vi "Create IResultHandler.vi"(8 "error in (no error)":errorcluster, 11 "IWampMessage":refnum<class "IWampMessage.lvclass">) -> (0 "error out":errorcluster, 3 "IResultHandler":refnum<class "IResultHandler.lvclass">)   [LabVIEW 2020, in "wamplv.lvlib"]
uses:
  wamplv.lvlib
  SerialisedMessages/JSONMessage/WampMessage JSON.lvclass
  SerialisedMessages/MsgPackMessage/WampMessage MsgPack.lvclass
  SerialisedMessages/IWampMessage/IWampMessage.lvclass
  ResultHandler JSON/ResultHandler JSON.lvclass
  ResultHandler MsgPack/ResultHandler MsgPack.lvclass
  C:/local/wamplv/Private/Requests/IGenericInternalMessage/IGenericInternalMessage.lvclass
  C:/local/wamplv/Private/Requests/IInternalMessage/IInternalMessage.lvclass
  C:/local/wamplv/Private/Requests/MessageReceivedHandlers/Result/IResultHandler/IResultHandler.lvclass
  C:/local/wamplv/Private/Requests/MessageReceivedHandlers/Result/ResultHandler JSON/ResultHandler JSON.lvclass
  C:/local/wamplv/Private/Requests/MessageReceivedHandlers/IJsonMessageHandler/IJsonMessageHandler.lvclass
  C:/local/wamplv/Private/Requests/MessageReceivedHandlers/Result/ResultHandler MsgPack/ResultHandler MsgPack.lvclass
  C:/local/wamplv/Private/Requests/MessageReceivedHandlers/IMsgPackMessageHandler/IMsgPackMessageHandler.lvclass
  IResultHandler/IResultHandler.lvclass
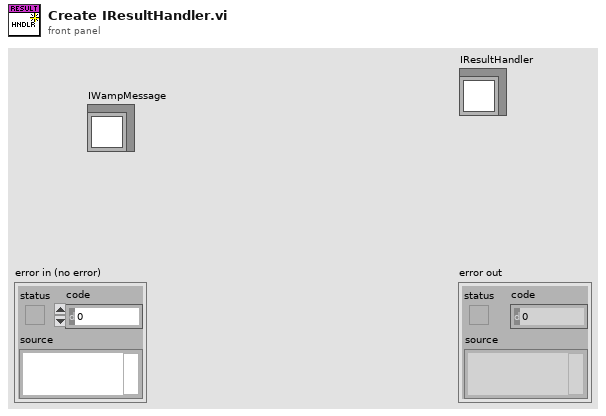
[diagram p1: front panel]
types:
  T1 = typedef "wamplv.lvlib/WAMP Client.lvclass/Serialisation.ctl" = enum16{"JSON", "MessagePack"}
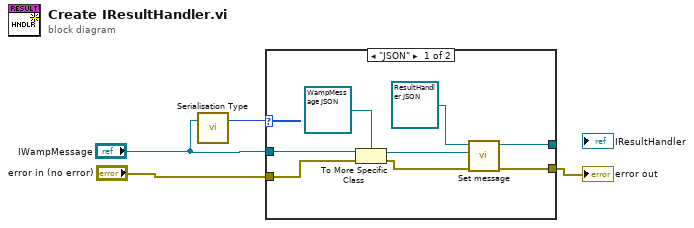
[diagram p0: block diagram]
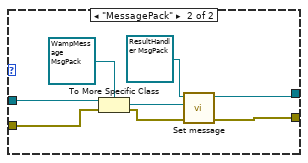
[diagram p2: hidden frame]
diagram:
  n1 = call-dynamic "Serialisation Type.vi"("IWampMessage in"="IWampMessage") -> ("Serialisation Type"=w4:T1)  [unwired: 2 in]
  n2 = case shown="\"JSON\"" w4 {
    tunnel: "IWampMessage" -> [w11 w18]
    tunnel: "error in (no error)" -> [w9 w17]
    tunnel: [w5 w12] -> _
    tunnel: [w6 w15] -> w2
    frame "JSON" {
      n3 = To More Specific Class(target class=refnum<class "WampMessage JSON.lvclass"> refnum ("wamplv.lvlib:JSONMessage.lvclass"), reference=w11, error in=w9) -> (specific class reference=w7:refnum<class "WampMessage JSON.lvclass">, error out=w6:errorcluster)
      n4 = call-dynamic "Set message.vi"("WampMessage JSON"=w7, "IMsgPackMessageHandler in"=refnum<class "ResultHandler JSON.lvclass"> refnum ("wamplv.lvlib:ResultHandler JSON.lvclass")) -> ("IMsgPackMessageHandler out"=w5:refnum<class "ResultHandler JSON.lvclass">)  [unwired: 9 in]
    }
    frame "MessagePack" {
      n5 = To More Specific Class(target class=refnum<class "WampMessage MsgPack.lvclass"> refnum ("wamplv.lvlib:MsgPackMessage.lvclass"), reference=w18, error in=w17) -> (specific class reference=w14:refnum<class "WampMessage MsgPack.lvclass">, error out=w15:errorcluster)
      n6 = call-dynamic "Set message.vi"("WampMessage MsgPack"=w14, "ResultHandler MsgPack in"=refnum<class "ResultHandler MsgPack.lvclass"> refnum ("wamplv.lvlib:ResultHandler MsgPack.lvclass")) -> ("ResultHandler MsgPack out"=w12:refnum<class "ResultHandler MsgPack.lvclass">)  [unwired: 9 in]
    }
  }
  "error out" <- w2
